vi "ex12.vi"() -> ()   [LabVIEW 2019]
panel:
  out "x/y":dbl
  out "x-y":dbl
  in  "y":dbl
  in  "x":dbl
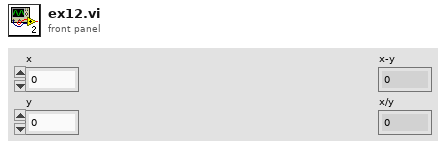
[diagram p1: front panel]
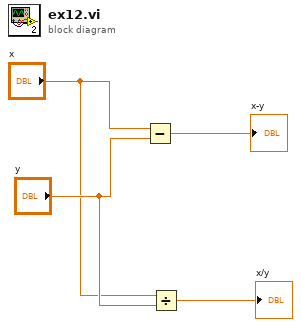
[diagram p0: block diagram]
diagram:
  n1 = Subtract(x="x", y="y") -> (x-y=→"x-y":dbl)
  n2 = Divide(x="x", y="y") -> (x/y=→"x/y":dbl)
